vi "Grating Number.vi"(8 "error in (no error)":errorcluster, 10 "Close VISA?":bool, 11 "VISA resource name":refnum<visa-resource-name>) -> (0 "error out":errorcluster, 2 "Grating being chosen":string, 3 "VISA resource name out":refnum<visa-resource-name>)   [LabVIEW 2009]
panel:
  out "return count":u32
  out "read buffer":string
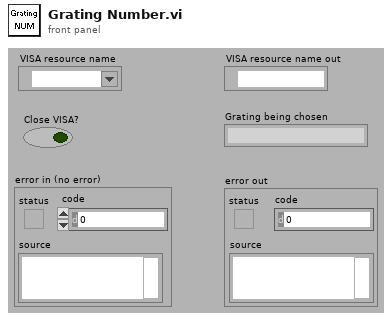
[diagram p1: front panel]
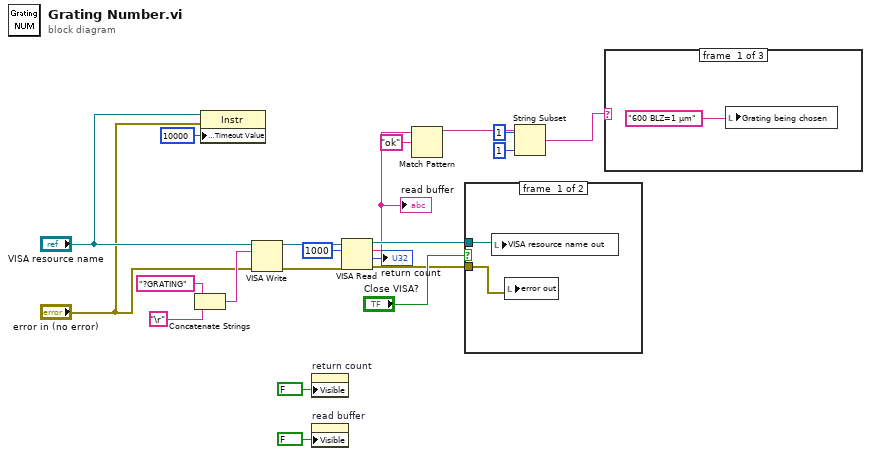
[diagram p0: block diagram]
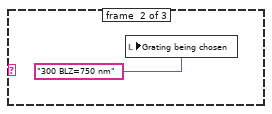
[diagram p2: hidden frame]
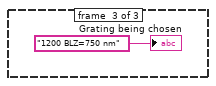
[diagram p3: hidden frame]
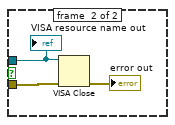
[diagram p4: hidden frame]
diagram:
  n1 = Concatenate Strings("?GRATING", "\r") -> (w20:string)
  n2 = property class="Instr"(reference="VISA resource name", error in="error in (no error)", "General Settings:Timeout Value"=u32 10000) -> ()  [unwired: 2 out]
  n3 = VISA Write(VISA resource name="VISA resource name", write buffer=w20, error in (no error)="error in (no error)") -> (VISA resource name out=w13:refnum<visa-resource-name>, error out=w12:errorcluster)  [unwired: 1 out]
  n4 = property on="return count" class="DigNum (strict)"("Visible"=FALSE) -> ()  [unwired: 2 in, 2 out]
  n5 = property on="read buffer" class="Str"("Visible"=FALSE) -> ()  [unwired: 2 in, 2 out]
  n6 = VISA Read(VISA resource name=w13, byte count=u32 1000, error in (no error)=w12) -> (VISA resource name out=w18:refnum<visa-resource-name>, read buffer=w16:string, return count=→"return count":u32, error out=w17:errorcluster)
  "read buffer" <- w16
  n7 = Match Pattern(string=w16, regular expression="ok") -> (before substring=w4:string)  [unwired: 4 out]
  n8 = case shown="False" "Close VISA?" {
    tunnel: w18 -> [w23 w26]
    tunnel: w17 -> [w22 w25]
    frame #0 {
      n9 = local write "VISA resource name out"(w23) -> ()
      n10 = local write "error out"(w22) -> ()
    }
    frame #1 {
      n11 = VISA Close(VISA resource name=w26, error in (no error)=w25) -> (error out=→"error out":errorcluster)
      "VISA resource name out" <- w26
    }
  }
  n12 = String Subset(string=w4, offset (0)=1, length (rest)=1 ("length (rest)")) -> (substring=w1:string)
  n13 = case shown="\"3\"" w1 {
    frame #0 {
      n14 = local write "Grating being chosen"("600 BLZ=1 µm") -> ()
    }
    frame #1 {
      n15 = local write "Grating being chosen"("300 BLZ=750 nm") -> ()
    }
    frame #2 {
      "Grating being chosen" <- "1200 BLZ=750 nm"
    }
  }
